vi "testing_readMeasurements_selfRecovery.vi"() -> ()   [LabVIEW 2015, in "Tausand AB1000.lvlib"]
uses:
  <instrlib>/Tausand AB1000/Tausand AB1000.lvlib
panel:
  out "último fallo":i32
  out "total mal":i32
  out "total ok":i16
  out "i":i32
  out "checksum ok?":bool
  out "chk":bool[](array[boolean])
  out "t":dbl[](array[numeric])
  out "min index(es)":i32
  out "min value":dbl
  out "max index(es)":i32
  out "max value":dbl
  in  "VISA resource name":refnum<visa-resource-name>
  out "time":dbl
  in  "iteraciones deseadas":i32
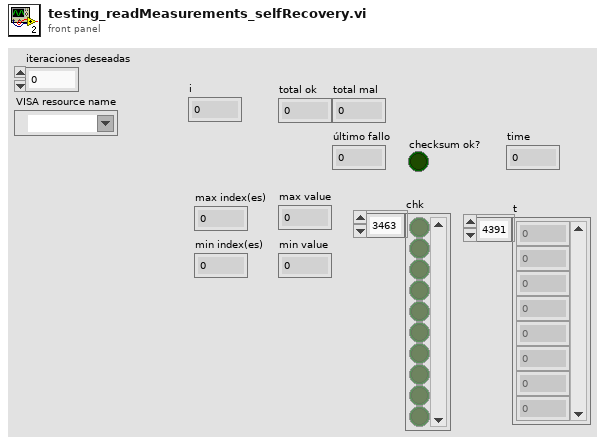
[diagram p1: front panel]
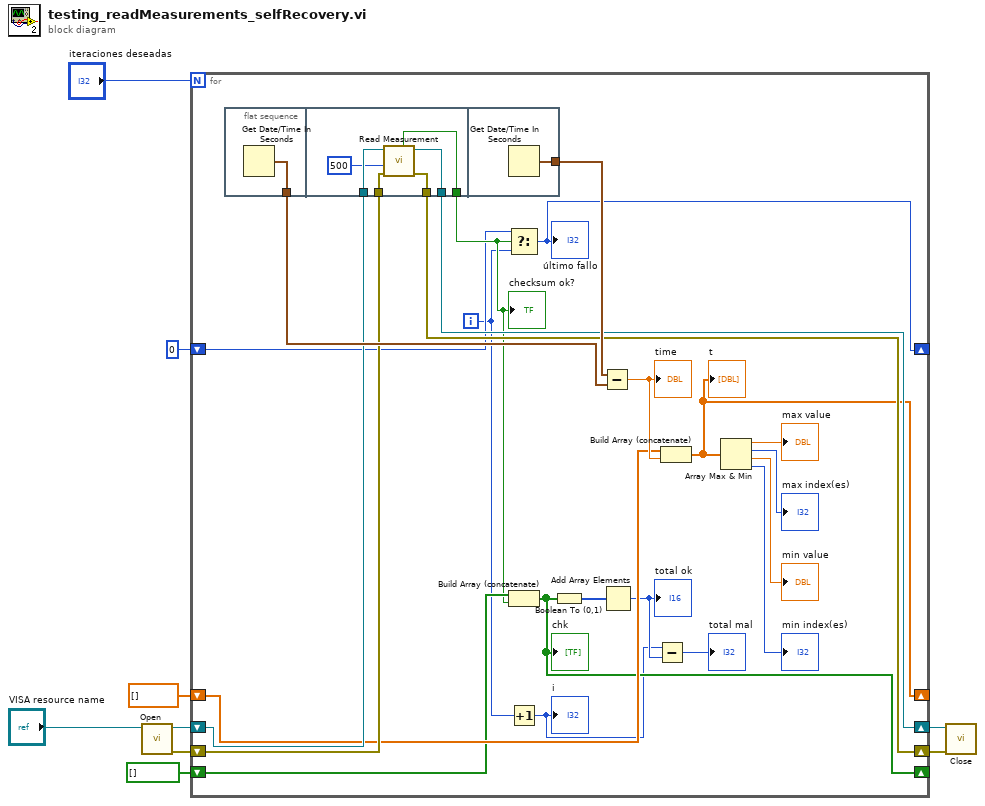
[diagram p0: block diagram]
diagram:
  n1 = call <instrlib>:"Open.vi"("VISA resource name"="VISA resource name") -> ("error out"=w6:errorcluster, "VISA resource name out"=w8:refnum<visa-resource-name>)  [unwired: 9 in]
  n2 = for {
    N: "iteraciones deseadas" -> [_]
    shift-right: [w28] -> w5
    shift-left: w6 -> [w29]
    shift-right: [w27] -> w4
    shift-left: w8 -> [w30]
    shift-right: [w20] -> _
    shift-left: dbl[] [] -> [w25]
    shift-right: [w17] -> _
    shift-left: bool[] [] -> [w19]
    shift-right: [w11] -> _
    shift-left: 0 ("f") -> [w12]
    i -> [w10]
    n3 = flat-sequence {
      tunnel: [w33] -> w31
      tunnel: w30 -> [w39]
      tunnel: w29 -> [w38]
      tunnel: [w37] -> w28
      tunnel: [w36] -> w27
      tunnel: [w35] -> w14
      tunnel: [w40] -> w32
      frame #0 {
        n4 = Get Date/Time In Seconds() -> (seconds since 1Jan1904=w33:timestamp)
      }
      frame #1 {
        n5 = call <instrlib>:"Read Measurement.vi"("error in (no error)"=w38, "read timeout (500 ms)"=u32 500, "VISA Refnum in"=w39) -> ("error out"=w37:errorcluster, "VISA Refnum out"=w36:refnum<visa-resource-name>, "checksum ok?"=w35:bool)  [unwired: 3 in, 3 out]
      }
      frame #2 {
        n6 = Get Date/Time In Seconds() -> (seconds since 1Jan1904=w40:timestamp)
      }
    }
    n7 = Select(t=w12, s=w14, f=w10) -> (s? t:f=w11:i32)
    "último fallo" <- w11
    n8 = Build Array (concatenate)(w19, w14) -> (w17:bool[])
    "chk" <- w17
    n9 = Increment(x=w10) -> (x+1=w13:i32)
    "i" <- w13
    n10 = Boolean To (0,1)(Boolean=w17) -> (0, 1=w18:i16[])
    n11 = Subtract(x=w32, y=w31) -> (x-y=w26:dbl)
    "time" <- w26
    n12 = Add Array Elements(numeric array=w18) -> (sum=w16:i16)
    "total ok" <- w16
    n13 = Subtract(x=w13, y=w16) -> (x-y=→"total mal":i32)
    n14 = Build Array (concatenate)(w25, w26) -> (w20:dbl[])
    "t" <- w20
    n15 = Array Max & Min(array=w20) -> (max value=→"max value":dbl, max index (indices)=→"max index(es)":i32, min value=→"min value":dbl, min index (indices)=→"min index(es)":i32)
    "checksum ok?" <- w14
  }
  n16 = call <instrlib>:"Close.vi"("error in (no error)"=w5, "VISA resource name"=w4) -> ()  [unwired: 9 in, 1 out]
